vi "Logging Trigger.vi"(8 "SampleDelay(in)":u32, 9 "Sample Rate (Hz)":dbl, 11 "Last Event mS":u32) -> (0 "Edge Output":bool, 3 "Last Event mS":u32, 4 "Elapsed mS":u32, 6 "SampleDelay":u32)   [LabVIEW 2021]
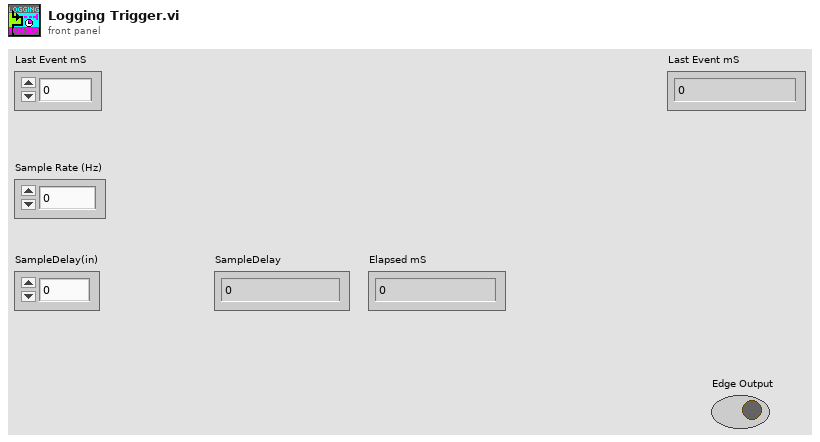
[diagram p1: front panel]
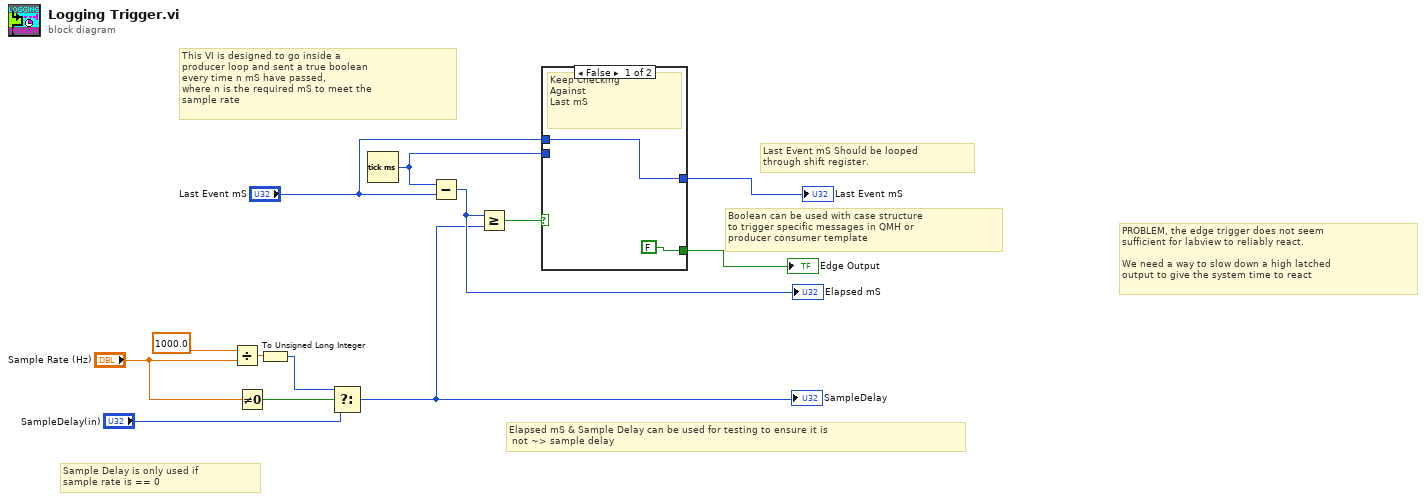
[diagram p0: block diagram]
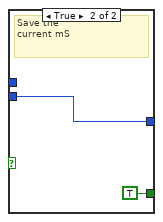
[diagram p2: hidden frame]
diagram:
  # "PROBLEM, the edge trigger does not seem \nsufficient for labview to reliably react.\n\nWe need a way to slow down a high latched \noutput to give the system time to react"
  # "Sample Delay is only used if\nsample rate is == 0"
  # "Elapsed mS & Sample Delay can be used for testing to ensure it is\n not ~> sample delay"
  # "Boolean can be used with case structure\nto trigger specific messages in QMH or \nproducer consumer template"
  # "This VI is designed to go inside a\nproducer loop and sent a true boolean\nevery time n mS have passed, \nwhere n is the required mS to meet the \nsample rate"
  # "Last Event mS Should be looped\nthrough shift register."
  n1 = Divide(x=1000.0, y="Sample Rate (Hz)") -> (x/y=w11:dbl)
  n2 = Not Equal To 0?(x="Sample Rate (Hz)") -> (x != 0?=w8:bool)
  n3 = To Unsigned Long Integer(number=w11) -> (unsigned 32bit integer=w7:u32)
  n4 = Select(t=w7, s=w8, f="SampleDelay(in)") -> (s? t:f=w1:u32)
  "SampleDelay" <- w1
  n5 = Tick Count (ms)() -> (millisecond timer value=w2:u32)
  n6 = Subtract(x=w2, y="Last Event mS") -> (x-y=w5:u32)
  "Elapsed mS" <- w5
  n7 = Greater Or Equal?(x=w5, y=w1) -> (x >= y?=w4:bool)
  n8 = case shown="False" w4 {
    tunnel: [w15 w17] -> w12
    tunnel: w2 -> [_ w17]
    tunnel: "Last Event mS" -> [w15 _]
    tunnel: [FALSE TRUE] -> w13
    frame False {
      # "Keep Checking\nAgainst\nLast mS"
    }
    frame True {
      # "Save the \ncurrent mS"
    }
  }
  "Last Event mS" <- w12
  "Edge Output" <- w13
